vi "Select OPC node IDs.vi"(11 "OPC Params":T5[](array[typedef]) {"data type" items=["Boolean"=1, "SByte"=2, "Byte"=3, "Int16"=4, "UInt16"=5, "Int32"=6, "UInt32"=7, "Int64"=8, "UInt64"=9, "Float"=10, "Double"=11, "String"=12, "DateTime"=13, "ByteString"=15, "Array of Boolean"=101, "Array of SByte"=102, "Array of Byte"=103, "Array of Int16"=104, "Array of UInt16"=105, "Array of Int32"=106, "Array of UInt32"=107, "Array of Int64"=108, "Array of UInt64"=109, "Array of Float"=110, "Array of Double"=111, "Array of String"=112, "Array of DateTime"=113, "Array of ByteString"=115, "Matrix of Boolean"=201, "Matrix of SByte"=202, "Matrix of Byte"=203, "Matrix of Int16"=204, "Matrix of UInt16"=205, "Matrix of Int32"=206, "Matrix of UInt32"=207, "Matrix of Int64"=208, "Matrix of UInt64"=209, "Matrix of Float"=210, "Matrix of Double"=211, "Matrix of String "=212, "Matrix of DateTime"=213, "Matrix of ByteString"=215]}) -> (1 "parameters":T1(array[cluster]), 2 "requests":T2[](array[typedef]) {"node status" items=["Good"=0, "Uncertain"=1073741824, "Uncertain_InitialValue"=1083310080, "Uncertain_LastUsableValue"=1083179008, "Uncertain_SensorNotAccurate"=1083375616, "Uncertain_EngineeringUnitsExceeded"=1083441152, "Bad"=2147483648, "Bad_NoCommunication"=2150694912, "Bad_NotReadable"=2151284736, "Bad_NotWritable"=2151350272, "Bad_OutOfRange"=2151415808, "Bad_WaitingForInitialData"=2150760448]}, 3 "node IDs":string[](array[string]))   [LabVIEW 2019, in "OPC addons.lvlib"]
uses:
  OPC addons.lvlib
  OPC tag.ctl
  <vilib>/OPCUA/controls/Data Type.ctl
  Access level.ctl
  Period.ctl
  <vilib>/OPCUA/controls/Write Variant Request.ctl
  <vilib>/OPCUA/controls/NodeId.ctl
  <vilib>/OPCUA/controls/Write Status.ctl
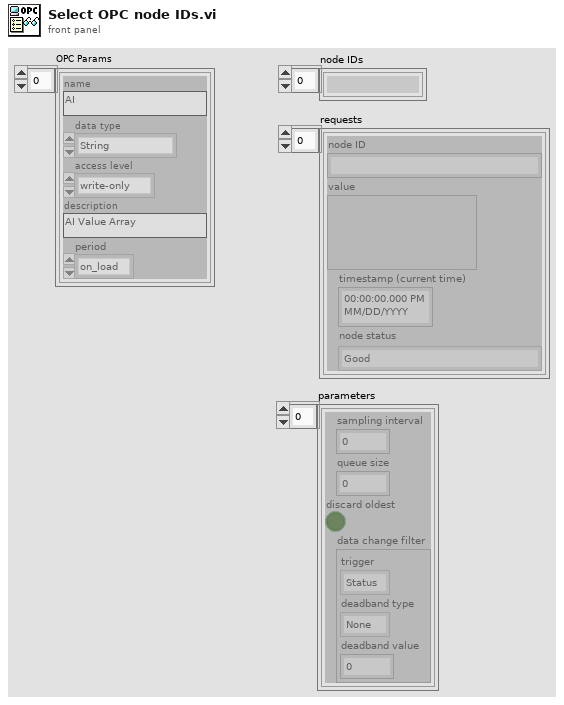
[diagram p1: front panel]
types:
  T1 = cluster{"sampling interval":dbl, "queue size":u32, "discard oldest":bool, "data change filter":cluster{"trigger":enum32{"Status", "StatusValue", "StatusValueTimestamp"}, "deadband type":enum32{"None", "Absolute", "Percent"}, "deadband value":dbl}}[]
  T2 = typedef "Write Variant Request.ctl" = cluster{"node ID":T3, "value":variant, "timestamp (current time)":timestamp, "node status":T4}
  T3 = typedef "NodeId.ctl" = string
  T4 = typedef "Write Status.ctl" = u32
  T5 = typedef "OPC addons.lvlib/OPC tag.ctl" = cluster{"name":string, "data type":T6, "access level":T7, "description":string, "period":T8}
  T6 = typedef "Data Type.ctl" = u16
  T7 = typedef "OPC addons.lvlib/Access level.ctl" = enum16{"none", "read-only", "write-only", "read/write"}
  T8 = typedef "OPC addons.lvlib/Period.ctl" = enum16{"on_load", "100 ms", "500 ms", "1 s"}
  T9 = cluster{"sampling interval":dbl, "queue size":u32, "discard oldest":bool, "data change filter":cluster{"trigger":enum32{"Status", "StatusValue", "StatusValueTimestamp"}, "deadband type":enum32{"None", "Absolute", "Percent"}, "deadband value":dbl}}
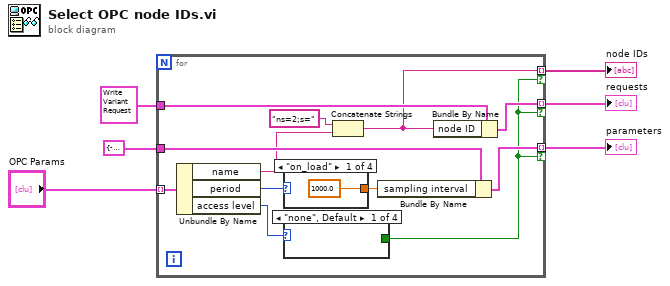
[diagram p0: block diagram]
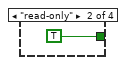
[diagram p2: hidden frame]
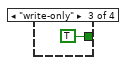
[diagram p3: hidden frame]
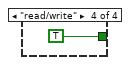
[diagram p4: hidden frame]
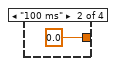
[diagram p5: hidden frame]
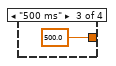
[diagram p6: hidden frame]
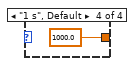
[diagram p7: hidden frame]
diagram:
  n1 = for {
    tunnel: [w18] -> w2 mode=indexing if=w7
    tunnel: T2 {"node ID"="", "value"=variant, "timestamp (current time)"=timestamp(0 s since 1904-01-01), "node status"=0} ("request") -> [w16]
    tunnel: "OPC Params" -> [w15] mode=indexing
    tunnel: T9 {"sampling interval"=-1.0, "queue size"=1, "discard oldest"=TRUE, "data change filter"={"trigger"=enum."StatusValue", "deadband type"=enum."None", "deadband value"=0.0}} ("monitoring parameters") -> [w14]
    tunnel: [w9] -> w3 mode=indexing if=w7
    tunnel: [w8] -> w1 mode=indexing if=w7
    n2 = Unbundle By Name(w15) -> ("name"=w11:string, "period"=w13:T8, "access level"=w10:T7)
    n3 = case shown="\"on_load\"" w13 {
      tunnel: [1000.0 ("sampling interval") 0.0 ("sampling interval") 500.0 ("sampling interval") 1000.0 ("sampling interval")] -> w12
      frame "on_load" {
      }
      frame "100 ms" {
      }
      frame "500 ms" {
      }
      frame "1 s", Default {
      }
    }
    n4 = case shown="\"none\", Default" w10 {
      tunnel: [_ TRUE TRUE TRUE] -> w7
      frame "none", Default {
      }
      frame "read-only" {
      }
      frame "write-only" {
      }
      frame "read/write" {
      }
    }
    n5 = Concatenate Strings("ns=2;s=" ("string"), w11) -> (w9:string)
    n6 = Bundle By Name(cluster=w14, "sampling interval"=w12) -> (w8:T9)
    n7 = Bundle By Name(cluster=w16, "node ID"=w9) -> (w18:T2)
  }
  "node IDs" <- w3
  "requests" <- w2
  "parameters" <- w1
